vi "VsEP Init Level Series.vi"(0 "STIMULUS":T2={"START dB re 1g/ms"=1, "STOP dB re 1g/ms"=20, "dB STEPSIZE"=0.0, "REP RATE (/sec)"=80.0, "Alternate Polarity"=TRUE, "Sampling Rate (Hz)"=5.0} {"dB STEPSIZE" format="%#_3g"; "START dB re 1g/ms" step=5}, 1 "Data Folder":path, 11 "error in (no error)":errorcluster) -> (8 "Max #Level":i32, 14 "Runtime":T1, 15 "error out":errorcluster)   [LabVIEW 2020]
uses:
  Typedefs/VsEP-Stimulus Control.ctl
  Typedefs/VsEP-Runtime Data.ctl
  epl-vi-lib/PXI DAQ VIs/DAQ Engine VIs/PXI Globals.vi
  epl-vi-lib/Utility VIs/Math VIs/Linear to dB (scalar).vi
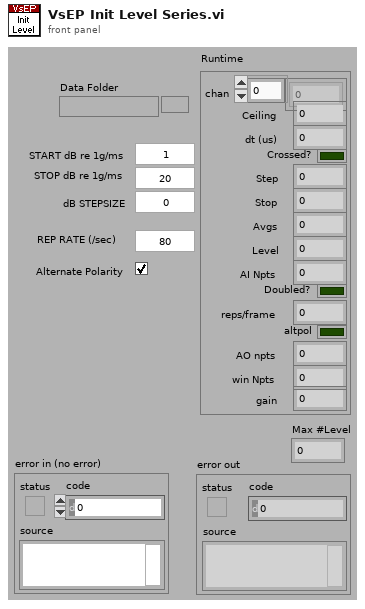
[diagram p1: front panel]
types:
  T1 = typedef "VsEP-Runtime Data.ctl" = cluster{"chan":i32[], "Ceiling":dbl, "dt (us)":dbl, "Crossed?":bool, "Step":dbl, "Stop":i32, "Avgs":i32, "Level":dbl, "AI Npts":i32, "Doubled?":bool, "reps/frame":i32, "altpol":bool, "AO npts":i32, "win Npts":i32, "gain":dbl}
  T2 = typedef "VsEP-Stimulus Control.ctl" = cluster{"START dB re 1g/ms":i32, "STOP dB re 1g/ms":i32, "dB STEPSIZE":sgl, "REP RATE (/sec)":dbl, "Alternate Polarity":bool, "Sampling Rate (Hz)":dbl}
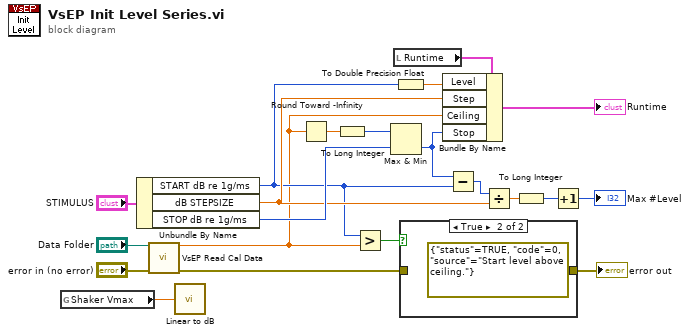
[diagram p0: block diagram]
diagram:
  n1 = global read "PXI Globals.vi" "Shaker Vmax"() -> (w2:dbl)
  n2 = Unbundle By Name("STIMULUS") -> ("START dB re 1g/ms"=w7:i32, "dB STEPSIZE"=w8:sgl, "STOP dB re 1g/ms"=w9:i32)
  n3 = call "VsEP Read Cal Data.vi"("Data Folder"="Data Folder", "error in (no error)"="error in (no error)") -> ("Sensitivity"=w6:dbl, "error out"=w4:errorcluster)  [unwired: 12 in]
  n4 = call-poly "Linear to dB.vi"("Linear"=w2) -> ()  [unwired: 1 out]
  n5 = Round Toward -Infinity(1:w6) -> (0:w1:dbl)
  n6 = To Long Integer(number=w1) -> (32bit integer=w16:i32)
  n7 = Greater?(x=w7, y=w6) -> (0:w5:bool)
  n8 = Max & Min(x=w16, y=w9) -> (min(x,y)=w13:i32)  [unwired: 1 out]
  n9 = local read "Runtime"() -> (w18:T1)
  n10 = To Double Precision Float(number=w7) -> (double precision float=w17:dbl)
  n11 = case shown="True" w5 {
    tunnel: [w22 errorcluster {"status"=TRUE, "code"=0, "source"="Start level above ceiling."} ("error out")] -> w3
    tunnel: w4 -> [w22 _]
    frame False {
    }
    frame True {
    }
  }
  "error out" <- w3
  n12 = Bundle By Name(cluster=w18, "Level"=w17, "Step"=w8, "Ceiling"=w6, "Stop"=w13) -> (→"Runtime":T1)
  n13 = Subtract(x=w13, y=w7) -> (x-y=w14:i32)
  n14 = Divide(x=w14, y=w8) -> (x/y=w12:sgl)
  n15 = To Long Integer(number=w12) -> (32bit integer=w11:i32)
  n16 = Increment(x=w11) -> (x+1=→"Max #Level":i32)
